vi "Rolling Average Umschaltung Anzeige.vi"(11 "error in (no error)":errorcluster caption="Fehler (Eingang, kein Fehler)", 13 "Aktion":enum16{"AK", "IAG Software"}(ring)) -> (3 "Aktuelle Messwerte":sgl[](array[numeric]), 4 "Messdaten":sgl[][](array[numeric]), 6 "Mittelwertdaten":sgl[][](array[numeric]), 8 "Deviation":sgl[](array[numeric]), 10 "Zeitstempeln":timestamp[](array[timestamp]), 15 "error out":errorcluster caption="Fehler (Ausgang)")   [LabVIEW 2020, in "Messdaten.lvlib"]
uses:
  Messdaten.lvlib
  Aktionen FGV Messdaten.ctl
  Seiten/FT-IR/Aktionen EVID-Codes.ctl
  Seiten/FT-IR/FT-IR.lvlib
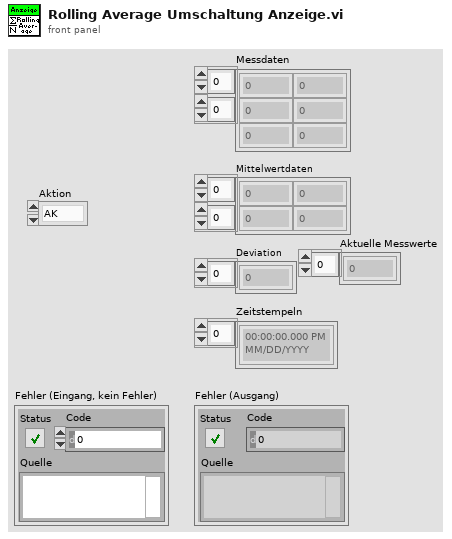
[diagram p1: front panel]
types:
  T1 = typedef "Messdaten.lvlib/Aktionen FGV Messdaten.ctl" = enum16{"lesen", "schreiben", "löschen", "Mittelwerte", "Komponente"}
  T2 = typedef "Messdaten.lvlib/Rolling Average Daten.ctl" = cluster{"RA aktuelle Messwerte":sgl[], "RA Messdaten":sgl[][], "RA Deviation":sgl[], "RA Zeitstempeln":timestamp[], "Rohwerte FTIR":sgl[][]}
  T3 = typedef "FT-IR.lvlib/Aktionen EVID-Codes.ctl" = enum16{"lesen", "setzen", "laden", "speichern", "1Hz/5Hz", "Smoothing", "Rolling Average"}
  T4 = typedef "FT-IR.lvlib/Rolling Average Settings.ctl" = cluster{"Average":u32, "Average via AK:":bool, "Average IAG Software:":bool}
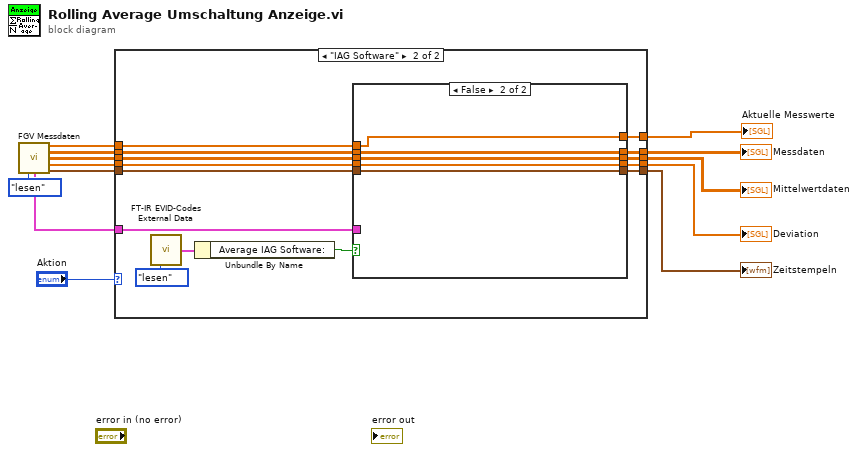
[diagram p0: block diagram]
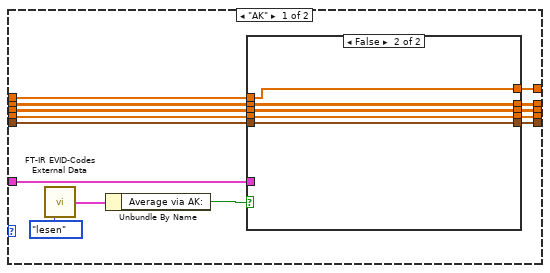
[diagram p2: hidden frame]
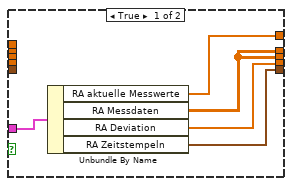
[diagram p3: hidden frame]
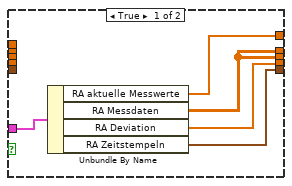
[diagram p4: hidden frame]
diagram:
  n1 = call "FGV Messdaten.vi"("Aktionen"=Aktionen_FGV_Messdaten."lesen") -> ("Aktuelle Messwerte"=w3:sgl[], "Messdaten"=w11:sgl[][], "Mittelwertdaten"=w9:sgl[][], "Deviation"=w7:sgl[], "Ausgangs-Cluster"=w12:T2, "Zeitstempeln"=w5:timestamp[])  [unwired: 6 in, 3 out]
  n2 = case shown="\"IAG Software\"" "Aktion" {
    tunnel: w12 -> [w27 w51]
    tunnel: w11 -> [w26 w50]
    tunnel: [w25 w49] -> w10
    tunnel: w9 -> [w24 w48]
    tunnel: [w23 w47] -> w8
    tunnel: w7 -> [w22 w46]
    tunnel: [w21 w45] -> w6
    tunnel: w5 -> [w20 w44]
    tunnel: [w19 w43] -> w4
    tunnel: w3 -> [w18 w42]
    tunnel: [w17 w41] -> w2
    frame "AK" {
      n3 = call "FT-IR EVID-Codes External Data.vi"("Aktionen"=Aktionen_EVID-Codes."lesen") -> ("Rolling Average Settings"=w16:T4)  [unwired: 9 in, 5 out]
      n4 = Unbundle By Name(w16) -> ("Average via AK:"=w14:bool)
      n5 = case shown="False" w14 {
        tunnel: w27 -> [w32 _]
        tunnel: w26 -> [_ w37]
        tunnel: [w28 w37] -> w25
        tunnel: w24 -> [_ w36]
        tunnel: [w28 w36] -> w23
        tunnel: w22 -> [_ w35]
        tunnel: [w31 w35] -> w21
        tunnel: w20 -> [_ w34]
        tunnel: [w30 w34] -> w19
        tunnel: [w29 w33] -> w17
        tunnel: w18 -> [_ w33]
        frame True {
          n6 = Unbundle By Name(w32) -> ("RA aktuelle Messwerte"=w29:sgl[], "RA Messdaten"=w28:sgl[][], "RA Deviation"=w31:sgl[], "RA Zeitstempeln"=w30:timestamp[])
        }
        frame False {
        }
      }
    }
    frame "IAG Software" {
      n7 = call "FT-IR EVID-Codes External Data.vi"("Aktionen"=Aktionen_EVID-Codes."lesen") -> ("Rolling Average Settings"=w40:T4)  [unwired: 9 in, 5 out]
      n8 = Unbundle By Name(w40) -> ("Average IAG Software:"=w38:bool)
      n9 = case shown="False" w38 {
        tunnel: w51 -> [w56 _]
        tunnel: w50 -> [_ w61]
        tunnel: [w52 w61] -> w49
        tunnel: w48 -> [_ w60]
        tunnel: [w52 w60] -> w47
        tunnel: w46 -> [_ w59]
        tunnel: [w55 w59] -> w45
        tunnel: w44 -> [_ w58]
        tunnel: [w54 w58] -> w43
        tunnel: [w53 w57] -> w41
        tunnel: w42 -> [_ w57]
        frame True {
          n10 = Unbundle By Name(w56) -> ("RA aktuelle Messwerte"=w53:sgl[], "RA Messdaten"=w52:sgl[][], "RA Deviation"=w55:sgl[], "RA Zeitstempeln"=w54:timestamp[])
        }
        frame False {
        }
      }
    }
  }
  "Messdaten" <- w10
  "Mittelwertdaten" <- w8
  "Deviation" <- w6
  "Zeitstempeln" <- w4
  "Aktuelle Messwerte" <- w2
